vi "Tilted Logistic Square Pulse Guess Parameters.vi"(8 "A_L":dbl, 9 "F Array":dbl[](array[numeric]), 10 "t Array":dbl[](array[numeric]), 11 "tr1, tr2, tf1, tf2":dbl[](array[numeric])) -> (3 "Guess Parameters":dbl[](array[numeric]))   [LabVIEW 2021, in "Fits.lvlib"]
uses:
  b030ed1a-ee8f-4b1c-8431-0d3fc4eb4993.vi
  c8742ba1-5fb7-4c70-9af5-f88f5e0edf1f.vi
  bef1792e-42da-4aa5-af31-1538c856ccfd.vi
  Fits.lvlib
panel:
  # "(tr1, tr2, tf1, tf2)"
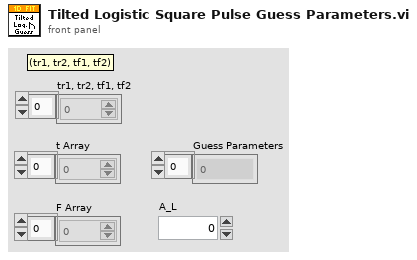
[diagram p1: front panel]
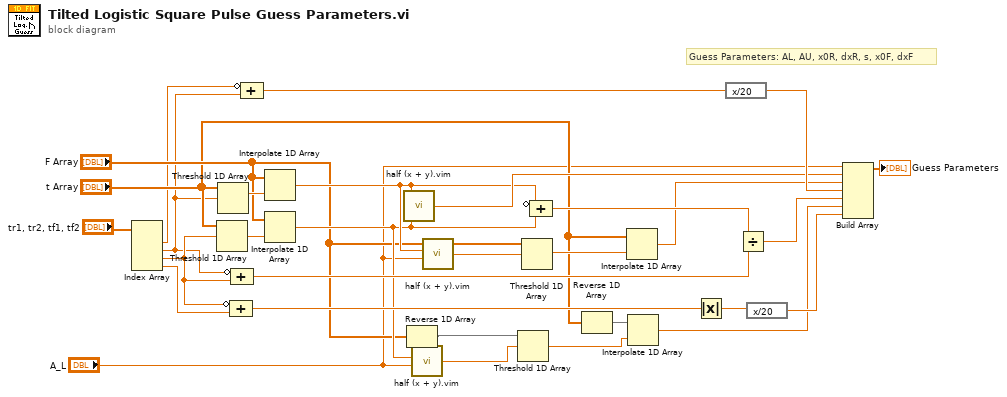
[diagram p0: block diagram]
diagram:
  # "Guess Parameters: AL, AU, x0R, dxR, s, x0F, dxF"
  n1 = Index Array(array="tr1, tr2, tf1, tf2") -> (element #1=w4:dbl, element #2=w3:dbl, element #3=w5:dbl, element #4=w6:dbl)  [unwired: 4 in]
  n2 = Threshold 1D Array(2:w5, 3:"t Array") -> (0:w26:dbl)  [unwired: 1 in]
  n3 = Threshold 1D Array(2:w3, 3:"t Array") -> (0:w27:dbl)  [unwired: 1 in]
  n4 = Compound Arithmetic op=ADD(invert w5, w6) -> (w21:dbl)
  n5 = Compound Arithmetic op=ADD(invert w3, w5) -> (w23:dbl)
  n6 = Compound Arithmetic op=ADD(invert w4, w3) -> (w2:dbl)
  n7 = Interpolate 1D Array(1:w27, 2:"F Array") -> (0:w16:dbl)
  n8 = Interpolate 1D Array(1:w26, 2:"F Array") -> (0:w14:dbl)
  n9 = call "half (x + y).vim"("y"=w14, "x"=w16) -> ("(x+y)/2"=w25:dbl)  [unwired: 4 in]
  n10 = Reverse 1D Array(array="F Array") -> (reversed array=w12:dbl[])
  n11 = call "half (x + y).vim"("y"="A_L", "x"=w14) -> ("(x+y)/2"=w11:dbl)  [unwired: 4 in]
  n12 = call "half (x + y).vim"("y"="A_L", "x"=w16) -> ("(x+y)/2"=w15:dbl)  [unwired: 4 in]
  n13 = Threshold 1D Array(2:w11, 3:w12) -> (0:w8:dbl)  [unwired: 1 in]
  n14 = Threshold 1D Array(2:w15, 3:"F Array") -> (0:w18:dbl)  [unwired: 1 in]
  n15 = Compound Arithmetic op=ADD(invert w16, w14) -> (w24:dbl)
  n16 = Reverse 1D Array(array="t Array") -> (reversed array=w9:dbl[])
  n17 = Interpolate 1D Array(1:w18, 2:"t Array") -> (0:w17:dbl)
  n18 = Interpolate 1D Array(1:w8, 2:w9) -> (0:w7:dbl)
  n19 = Absolute Value(x=w21) -> (abs(x)=w19:dbl)
  n20 = expression code="x/20"(w2) -> (w30:dbl)
  n21 = Divide(x=w24, y=w23) -> (x/y=w22:dbl)
  n22 = expression code="x/20"(w19) -> (w20:dbl)
  n23 = Build Array("A_L", w25, w17, w30, w22, w7, w20) -> (→"Guess Parameters":dbl[])
